vi "UDP서버장난감.vi"() -> ()   [LabVIEW 2018]
uses:
  <vilib>/Utility/tcp.llb/UDP Multicast Write-Only Open.vi
panel:
  out "날짜/시간 문자열":string
  in  "시간 전달":bool
  in  "값 전달":cluster{"aaa":bool, "bbb":bool, "ccc":bool}
  in  "정지":bool
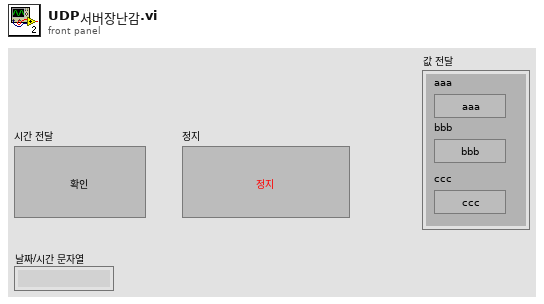
[diagram p1: front panel]
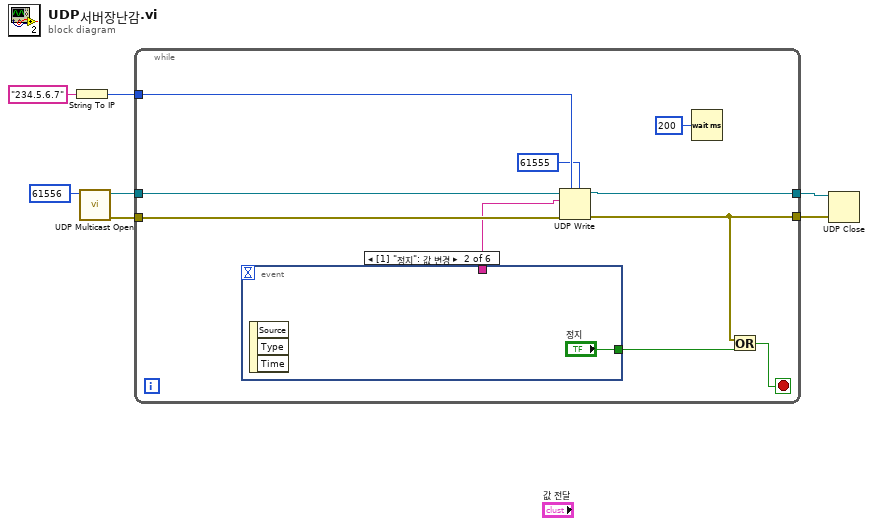
[diagram p0: block diagram]
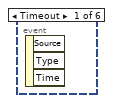
[diagram p2: hidden frame]
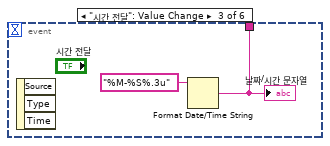
[diagram p3: hidden frame]
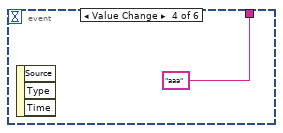
[diagram p4: hidden frame]
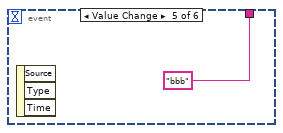
[diagram p5: hidden frame]
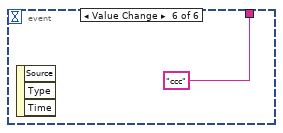
[diagram p6: hidden frame]
diagram:
  n1 = String To IP(1:"234.5.6.7" ("이름")) -> (0:w2:u32)
  n2 = call-poly <vilib>:"UDP Multicast Open.vi"("port"=u16 61556 ("포트")) -> ("error out"=w5:errorcluster, "connection ID"=w7:refnum<k16>)  [unwired: 9 in]
  n3 = while {
    tunnel: w7 -> [w17]
    tunnel: [w16] -> w6
    tunnel: w5 -> [w10]
    tunnel: [w13] -> w4
    tunnel: w2 -> [w15]
    stop <- w12 stop-if-true
    n4 = event shown="[1] \"정지\": 값 변경" {
      selector: _ -> [_ _ _ _ _ _]
      dyn-events: _ -> [_ _ _ _ _ _]
      timeout: _ -> [_ _ _ _ _ _]
      tunnel: [_ _ w19 "aaa" "bbb" "ccc"] -> w9
      tunnel: [_ "정지" _ _ _ _] -> w8
      event Timeout {
        n5 = event-data() -> ()  [unwired: 1 in, 3 out]
      }
      event "정지": Value Change {
        n6 = event-data() -> ()  [unwired: 1 in, 3 out]
      }
      event "시간 전달": Value Change {
        n7 = event-data() -> ()  [unwired: 1 in, 3 out]
        n8 = Format Date/Time String(time format string (%c)="%M-%S%.3u" ("시간 포맷 문자열 (%c)")) -> (date/time string=w19:string)  [unwired: 2 in]
        "날짜/시간 문자열" <- w19
      }
      event "값 전달.aaa": Value Change {
        n9 = event-data() -> ()  [unwired: 1 in, 3 out]
      }
      event "값 전달.bbb": Value Change {
        n10 = event-data() -> ()  [unwired: 1 in, 3 out]
      }
      event "값 전달.ccc": Value Change {
        n11 = event-data() -> ()  [unwired: 1 in, 3 out]
      }
    }
    n12 = UDP Write(address=w15, port or service name=u16 61555 ("포트 또는 서비스 이름"), connection ID=w17, data in=w9, 8:w10) -> (error out=w13:errorcluster, 3:w16:refnum<k16>)  [unwired: 1 in]
    n13 = Wait (ms)(milliseconds to wait=u32 200 ("대기 시간 (ms)")) -> ()  [unwired: 1 out]
    n14 = Or(x=w13, y=w8) -> (x .or. y?=w12:bool)
  }
  n15 = UDP Close(connection ID=w6, 8:w4) -> ()  [unwired: 2 out]
